vi "Exception Classic Error Throw.vi"(11 "error in (no error)":errorcluster) -> (4 "thrown":bool, 15 "error out":errorcluster)   [LabVIEW 2015, in "LV Exceptions v1.lvlib" / "Exception Classic Error.lvclass"]
doc: "Converst traditional error to exception. Exception is thrown by being forwarded in the error cluster."
uses:
  Exception Classic Error.lvclass
  Exception/Public/Exception Error Code.ctl
  Exception Classic Error.lvclass/Exception Classic Error.ctl
  <vilib>/Utility/error.llb/DialogType.ctl
  Exception/Exception.lvclass/Exception.ctl
  <vilib>/Utility/error.llb/Trim Whitespace.vi
  Exception/Exception.lvclass
panel:
  in  "Exception Classic Error":refnum<class "Exception Classic Error.lvclass">
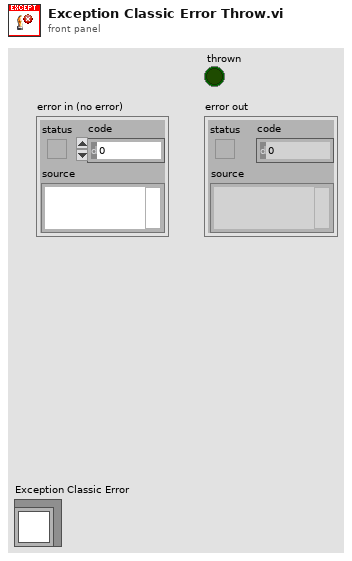
[diagram p1: front panel]
types:
  T1 = typedef "LV Exceptions v1.lvlib/Exception.lvclass/Exception Error Code.ctl" = i32
  T2 = typedef "DialogType.ctl" = u16
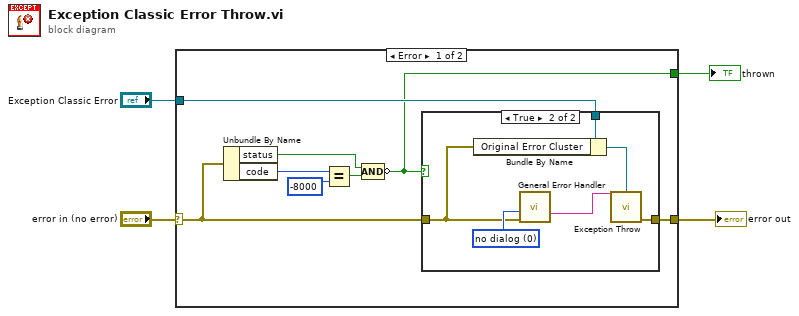
[diagram p0: block diagram]
diagram:
  n1 = case shown="Error" "error in (no error)" {
    selector: "error in (no error)" -> [w6 w20]
    tunnel: [w12 w20] -> w3
    tunnel: "Exception Classic Error" -> [w11 _]
    tunnel: [w5 _] -> w1
    frame Error {
      n2 = Unbundle By Name(w6) -> ("status"=w7:bool, "code"=w10:i32)
      n3 = Equal?(x=w10, y=T1 -8000) -> (x = y?=w8:bool)
      n4 = Compound Arithmetic op=AND(w7, w8) -> (invert w5:bool)
      n5 = case shown="True" w5 {
        tunnel: [w13 w19] -> w12
        tunnel: w11 -> [_ w18]
        tunnel: w6 -> [w13 w14]
        frame False {
        }
        frame True {
          w16 = T2 0 items=["no dialog", "OK message", "continue or stop message", "OK message + warnings", "continue/stop + warnings"] ("type of dialog (OK msg:1)")
          n6 = Bundle By Name(cluster=w18, "Original Error Cluster"=w14) -> (w17:refnum<class "Exception Classic Error.lvclass">)
          n7 = call <vilib>:"General Error Handler.vi"("type of dialog (OK msg:1)"=w16, "error in (no error)"=w14) -> ("message"=w15:string)  [unwired: 9 in, 4 out]
          n8 = call "Exception Throw.vi"("message"=w15, "Exception in"=w17) -> ("error out"=w19:errorcluster)  [unwired: 13 in]
        }
      }
    }
    frame No Error {
    }
  }
  "error out" <- w3
  "thrown" <- w1
